vi "Rectangularity Score.vi"(9 "Height":dbl, 10 "Width":dbl, 11 "Area":dbl) -> (3 "Score":dbl)   [LabVIEW 2025]
doc: "Use coverage of the bounding box to score higher on rectangles and lower on other shapes.\n\nPerfect rectangle scores 100.\nLess area coverage scores lower, proportionally.\n\nExpected to be used with vision. None of the inputs are expected to be negative."
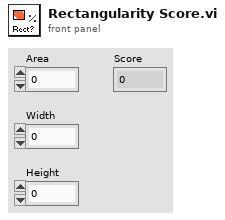
[diagram p1: front panel]
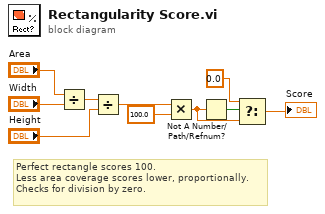
[diagram p0: block diagram]
diagram:
  # "Perfect rectangle scores 100.\nLess area coverage scores lower, proportionally.\nChecks for division by zero."
  n1 = Divide(x="Area", y="Width") -> (x/y=w7:dbl)
  n2 = Divide(x=w7, y="Height") -> (x/y=w6:dbl)
  n3 = Multiply(x=w6, y=100.0) -> (x*y=w3:dbl)
  n4 = Not A Number/Path/Refnum?(number/path/refnum=w3) -> (NaN/Path/Refnum?=w4:bool)
  n5 = Select(t=0.0 ("y"), s=w4, f=w3) -> (s? t:f=→"Score":dbl)
